vi "Get Root Path.vi"() -> (3 "Root Path":path=path "C:/PAS Circulation Tester")   [LabVIEW 2015]
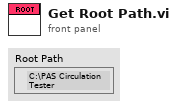
[diagram p1: front panel]
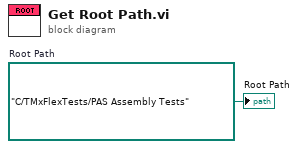
[diagram p0: block diagram]
diagram:
  w1 = path "C:/TMxFlexTests/PAS Assembly Tests"  # Root Path
  "Root Path" <- w1
